vi "Data Viewer.vi"() -> ()   [LabVIEW 2018]
uses:
  <vilib>/drjdpowell/SQLite Library/SQL Connection/Open (path).vi
  <vilib>/drjdpowell/SQLite Library/SQL Connection/Open (string).vi
  <vilib>/AdvancedString/Path To Command Line String.vi
  <vilib>/drjdpowell/SQLite Library/SQL Connection/Execute SQL.vi
  <vilib>/drjdpowell/SQLite Library/SQL Connection/Connection.lvclass
  <vilib>/drjdpowell/SQLite Library/SQLite.lvlib
panel:
  in  "Model":enum32{"ME 79", "ME 74"}(radio)
  in  "Get Data":bool
  in  "To":timestamp format="%<%H:%M:%S\n%Y/%m/%d>T"
  in  "From":timestamp format="%<%H:%M:%S\n%Y/%m/%d>T"
  in  "Search":bool
  in  "Scan Data Matrix":string
  in  "Exit":bool
  out "Data":string[][](table)
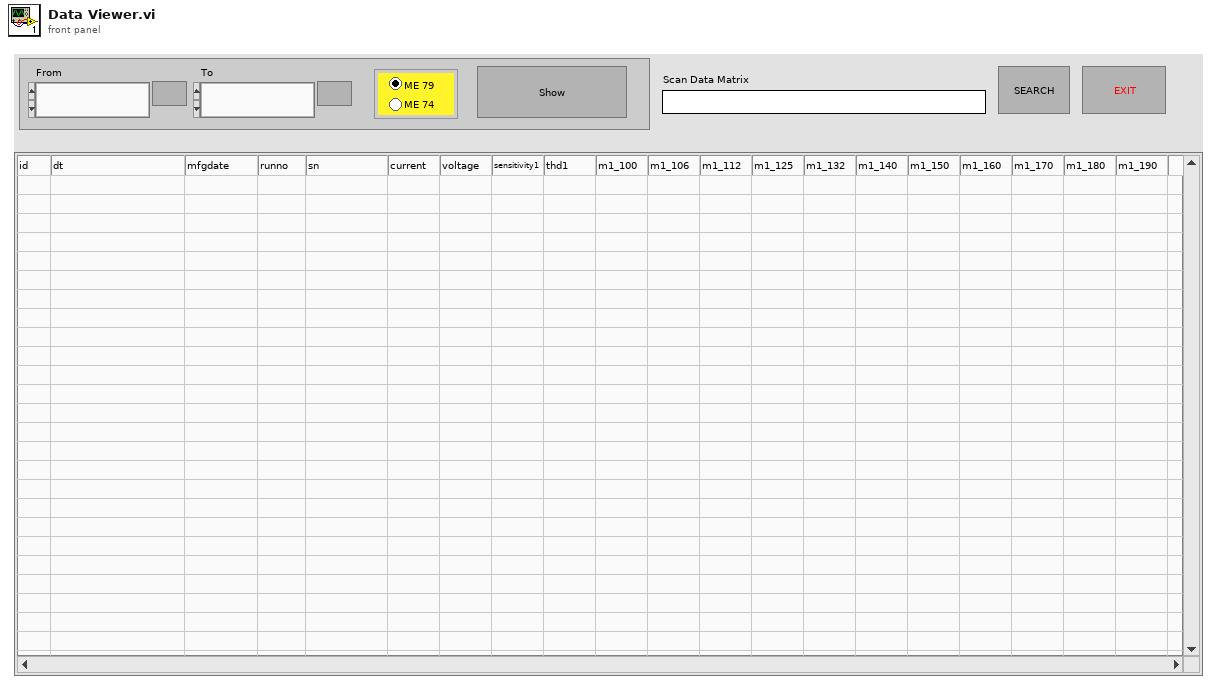
[diagram p1: front panel]
types:
  T1 = enum16{"New or existing", "Existing", "Read only"}
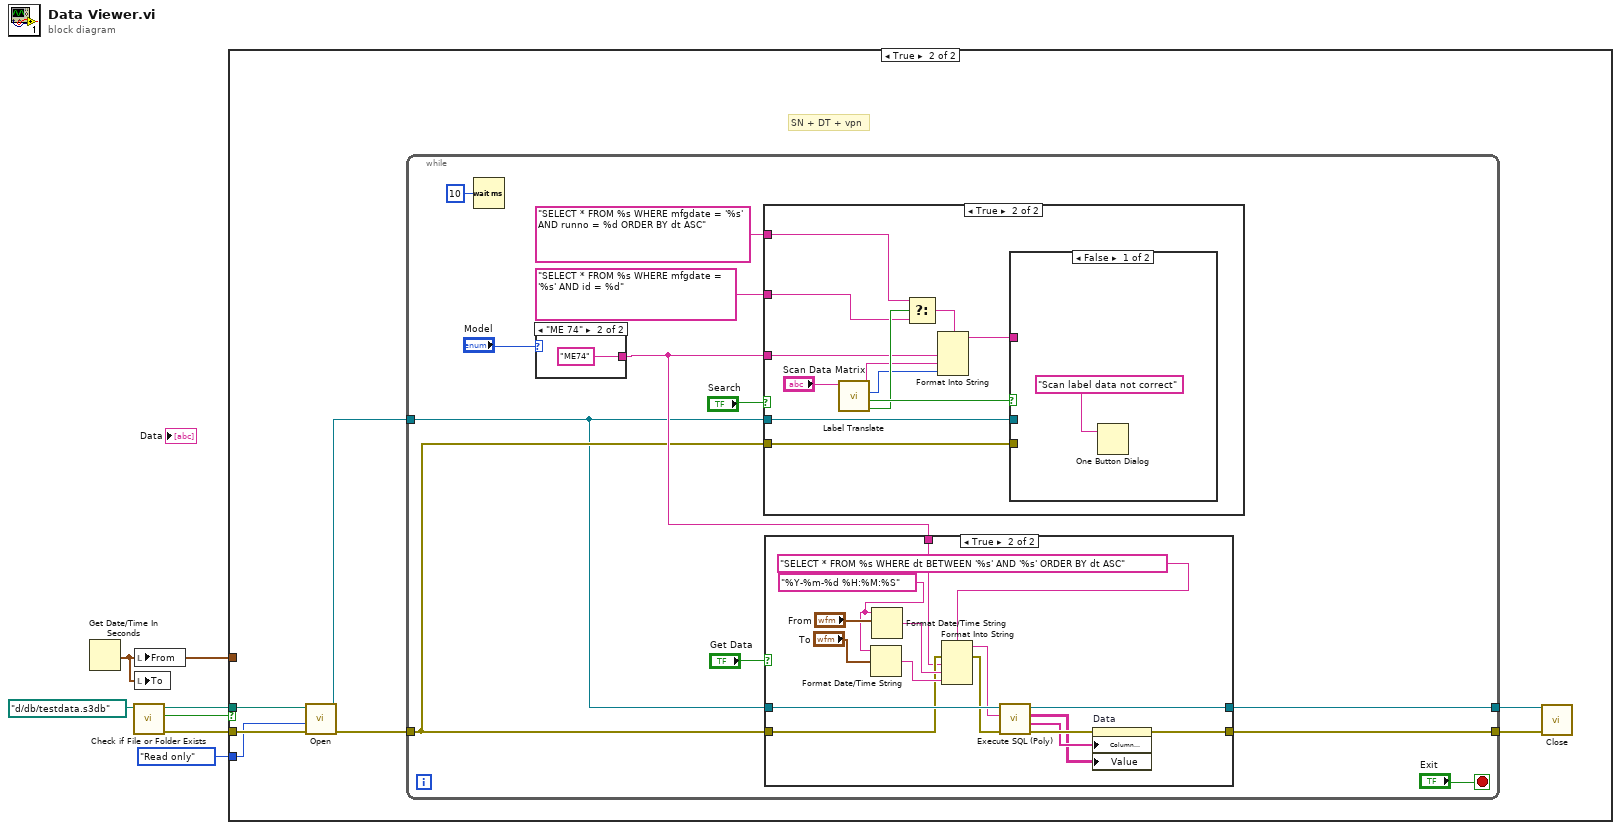
[diagram p0: block diagram]
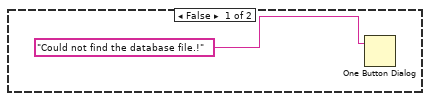
[diagram p2: hidden frame]
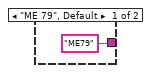
[diagram p3: hidden frame]
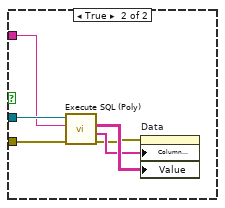
[diagram p5: hidden frame]
diagram:
  n1 = Get Date/Time In Seconds() -> (seconds since 1Jan1904=w1:timestamp)
  n2 = call <vilib>:"Check if File or Folder Exists.vi"("path"=path "d:/db/testdata.s3db" ("base path")) -> ("error out"=w4:errorcluster, "file or folder exists?"=w6:bool, "dup path"=w5:path)  [unwired: 8 in]
  n3 = local write "From"(w1) -> ()
  n4 = local write "To"(w1) -> ()
  n5 = case shown="True" w6 {
    tunnel: w5 -> [_ w10]
    tunnel: w4 -> [_ w12]
    tunnel: T1."Read only" ("File Option") -> [_ w11]
    tunnel: w1 -> [_ _]
    frame False {
      n6 = One Button Dialog(message="Could not find the database file.!") -> ()  [unwired: 1 in, 1 out]
    }
    frame True {
      # "SN + DT + vpn"
      n7 = call-poly <vilib>:"Open.vi"("error in (no error)"=w12, "File Option"=w11, "db file"=w10) -> ("error out"=w9:errorcluster, "SQLite Connection"=w8:refnum<class "Connection.lvclass">)  [unwired: 7 in]
      n8 = while {
        tunnel: [w24] -> w14
        tunnel: [w23] -> w13
        tunnel: w9 -> [w16]
        tunnel: w8 -> [w15]
        stop <- "Exit" stop-if-true
        n9 = Wait (ms)(milliseconds to wait=u32 10) -> ()  [unwired: 1 out]
        n10 = case shown="\"ME 74\"" "Model" {
          tunnel: ["ME79" "ME74"] -> w17
          frame "ME 79", Default {
          }
          frame "ME 74" {
          }
        }
        n11 = case shown="True" "Search" {
          tunnel: "SELECT * FROM %s WHERE mfgdate = '%s' AND runno = %d ORDER BY dt ASC" -> [_ w37]
          tunnel: "SELECT * FROM %s WHERE mfgdate = '%s' AND id = %d" -> [_ w36]
          tunnel: w15 -> [_ w32]
          tunnel: w16 -> [_ w31]
          tunnel: w17 -> [_ w29]
          frame False {
          }
          frame True {
            n12 = call "Label Translate.vi"("String In"="Scan Data Matrix") -> ("Test Result"=w38:bool, "Label OK"=w39:bool, "SN or ID"=w34:i32, "DTandShift"=w30:string)  [unwired: 7 in]
            n13 = Select(t=w37, s=w38, f=w36) -> (s? t:f=w35:string)
            n14 = Format Into String(format string=w35, w29, w30, w34) -> (resulting string=w33:string)  [unwired: 2 in, 1 out]
            n15 = case shown="False" w39 {
              tunnel: w33 -> [_ w46]
              tunnel: w32 -> [_ w47]
              tunnel: w31 -> [_ w45]
              frame False {
                n16 = One Button Dialog(message="Scan label data not correct") -> ()  [unwired: 1 in, 1 out]
              }
              frame True {
                n17 = call-poly <vilib>:"Execute SQL (Poly).vi"("error in (no error)"=w45, "SQL"=w46, "SQLite Connection in"=w47) -> ("error out"=w42:errorcluster, "Column Names"=w43:string[], "Result Set"=w44:string[][])  [unwired: 5 in, 1 out]
                n18 = property on="Data" class="Tbl (strict)"(error in=w42, "Column Headers[]"=w43, "Value"=w44) -> ()  [unwired: 1 in, 2 out]
              }
            }
          }
        }
        n19 = case shown="True" "Get Data" {
          tunnel: w16 -> [w49 w59]
          tunnel: w15 -> [w48 w63]
          tunnel: [w49 w54] -> w24
          tunnel: [w48 w53] -> w23
          tunnel: w17 -> [_ w50]
          frame False {
          }
          frame True {
            w52 = "%Y-%m-%d %H:%M:%S" ("time format string (%c)")
            n20 = Format Date/Time String(time format string (%c)=w52, seconds (now)="To") -> (date/time string=w61:string)  [unwired: 1 in]
            n21 = Format Date/Time String(time format string (%c)=w52, seconds (now)="From") -> (date/time string=w62:string)  [unwired: 1 in]
            n22 = Format Into String(format string="SELECT * FROM %s WHERE dt BETWEEN '%s' AND '%s' ORDER BY dt ASC", error in=w59, w50, w62, w61) -> (resulting string=w60:string, error out=w58:errorcluster)  [unwired: 1 in]
            n23 = call-poly <vilib>:"Execute SQL (Poly).vi"("error in (no error)"=w58, "SQL"=w60, "SQLite Connection in"=w63) -> ("error out"=w57:errorcluster, "Column Names"=w56:string[], "Result Set"=w55:string[][], "SQLite Connection"=w53:refnum<class "Connection.lvclass">)  [unwired: 5 in]
            n24 = property on="Data" class="Tbl (strict)"(error in=w57, "Column Headers[]"=w56, "Value"=w55) -> (error out=w54:errorcluster)  [unwired: 1 in, 1 out]
          }
        }
      }
      n25 = call-dynamic "Close.vi"("error in (no error)"=w14, "SQLite Connection in"=w13) -> ()  [unwired: 9 in, 1 out]
    }
  }
